vi "Stop Song.vi"(0 "reference in":refnum<class "MusicPlayer.lvclass">, 11 "Error In":errorcluster) -> (4 "reference out":refnum<class "MusicPlayer.lvclass">, 15 "Error Out":errorcluster)   [LabVIEW 2022 SP3, in "MusicPlayer.lvclass"]
uses:
  MusicPlayer.lvclass
  MusicPlayer.lvclass/MusicPlayer.ctl
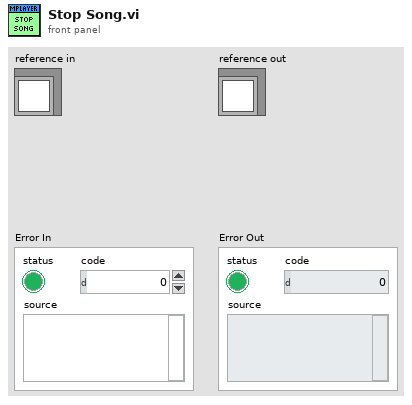
[diagram p1: front panel]
types:
  T1 = typedef "MusicPlayer.lvclass/ObjectAttributes.ctl" = cluster{"MediaPlayer":refnum<k7>, "Playlist":path[], "Index":u32}
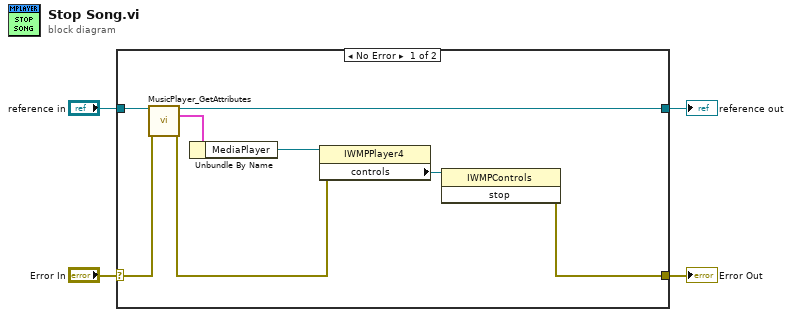
[diagram p0: block diagram]
diagram:
  n1 = case shown="No Error" "Error In" {
    selector: "Error In" -> [w12 w14]
    tunnel: [w6 w14] -> w3
    tunnel: [w9 w13] -> w1
    tunnel: "reference in" -> [w10 w13]
    frame No Error {
      n2 = call "MusicPlayer_GetAttributes.vi"("reference in"=w10, "error in (no error)"=w12) -> ("reference out"=w9:refnum<class "MusicPlayer.lvclass">, "Data"=w11:T1, "error out"=w5:errorcluster)  [unwired: 10 in, 1 out]
      n3 = Unbundle By Name(w11) -> ("MediaPlayer"=w8:refnum<k7>)
      n4 = property class="IWMPPlayer4"(reference=w8, error in=w5) -> ("controls"=w7:refnum<k7>)  [unwired: 2 out]
      n5 = invoke class="IWMPControls" method="stop"(reference=w7) -> (error out=w6:errorcluster)  [unwired: 2 in, 2 out]
    }
    frame Error {
    }
  }
  "Error Out" <- w3
  "reference out" <- w1
